vi "publishStatus.vi"(8 "error in (no error)":errorcluster, 10 "status":T1, 11 "Monochromator in":refnum<class "Monochromator.lvclass">) -> (0 "error out":errorcluster, 3 "Monochromator out":refnum<class "Monochromator.lvclass">)   [LabVIEW 2016, in "Monochromator.lvclass"]
uses:
  Monochromator.lvclass
  Typedefs/DeviceStatus.ctl
  Monochromator.lvclass/Monochromator.ctl
  MonoPubSubData/MonoPubSubData.lvclass/MonoPubSubData.ctl
  MonoPubSubData/MonoPubSubData.lvclass
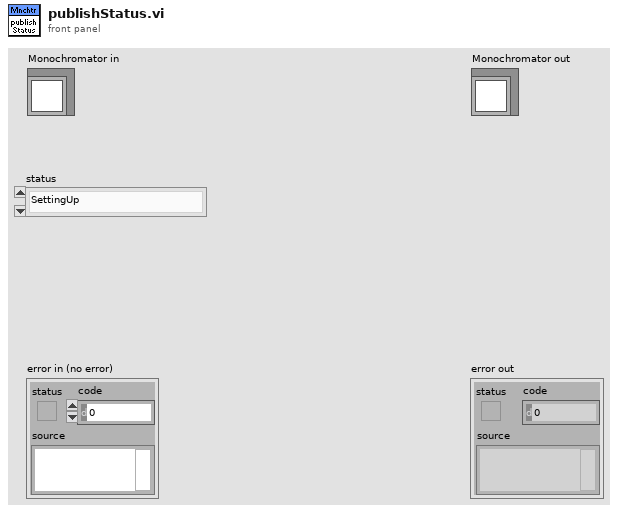
[diagram p1: front panel]
types:
  T1 = typedef "DeviceStatus.ctl" = enum16{"SettingUp", "Ready", "Offline", "Fault"}
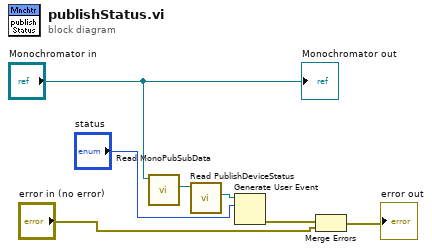
[diagram p0: block diagram]
diagram:
  n1 = call "Read MonoPubSubData.vi"("Monochromator in"="Monochromator in") -> ("MonoPubSubData.lvclass"=w4:refnum<class "MonoPubSubData.lvclass">)  [unwired: 8 in, 2 out]
  n2 = call "Read PublishDeviceStatus.vi"("MonoPubSubData in"=w4) -> ("PublishDeviceStatus"=w5:refnum<user-event>)  [unwired: 8 in, 2 out]
  n3 = Generate User Event(user event=w5, event data cluster="status") -> (error out=w3:errorcluster)  [unwired: 2 in, 1 out]
  n4 = Merge Errors(w3, "error in (no error)") -> (→"error out":errorcluster)
  "Monochromator out" <- "Monochromator in"
